vi "SP Retrieve Key Array for Config.vi"(8 "error in (no error)":errorcluster, 9 "Datasheets":T33, 10 "Key Array In":T34, 11 "Connection Refnum":T1) -> (0 "error out":errorcluster, 2 "S Parameter Test Parameters":T2={"Stimulus"={"Use Instrument Settings"=FALSE, "Blank Frequencies"=FALSE, "Sweep Type"=enum."Linear", "Sweep"={"Fstart"=500.0, "Fstop"=1500.0, "Units"=enum."MHz", "Points"=2}, "Power (dBm)"=999.0, "IFBW (Hz)"=-1.0, "Sweep Time (s)"=-1.0, "Calibration"={"State"=FALSE, "String"=""}}, "Measurement"={"Auto Select"=TRUE, "Data Source"=enum."VNA", "Ports"=2, "Parameters"=[]}, "De-Embed"={"De-Embed"=FALSE, "Adapters"=[]}, "Display"={"Lock Control"=FALSE, "Retain Settings"=TRUE, "Formatted Data"=FALSE, "Plot Orientation"=enum."Single", "Plot Controls"=[{"Trace Orientation"=enum."Overlay", "Frequency"={"Change Frequency"=FALSE, "Start"=500.0, "Stop"=1500.0, "Units"=enum."MHz"}, "Markers"=[], "Traces"=[]}, {"Trace Orientation"=enum."Overlay", "Frequency"={"Change Frequency"=FALSE, "Start"=500.0, "Stop"=1500.0, "Units"=enum."MHz"}, "Markers"=[], "Traces"=[]}, {"Trace Orientation"=enum."Overlay", "Frequency"={"Change Frequency"=FALSE, "Start"=500.0, "Stop"=1500.0, "Units"=enum."MHz"}, "Markers"=[], "Traces"=[]}, {"Trace Orientation"=enum."Overlay", "Frequency"={"Change Frequency"=FALSE, "Start"=500.0, "Stop"=1500.0, "Units"=enum."MHz"}, "Markers"=[], "Traces"=[]}]}, "Limits"=[], "Filter Limits"=[]} {"Filter Limits"."Parameter"."Stimulus Port" min=1 step=1; "Filter Limits"."Parameter"."Response Port" min=1 step=1; "Filter Limits"."Passband"."Bandwidth Attn" format="%.3g"; "Filter Limits"."Passband"."Stop/Span" format="%.3g"; "Filter Limits"."Passband"."Start/Center" format="%.3g"; "Measurement"."Parameters"."Channel" min=0 max=32 step=1; "Measurement"."Parameters"."Parameter"."Stimulus Port" min=1 step=1; "Measurement"."Parameters"."Parameter"."Response Port" min=1 step=1; "Limits"."Parameter"."Stimulus Port" min=1 step=1; "Limits"."Parameter"."Response Port" min=1 step=1; "Stimulus"."Sweep Time (s)" format="%.3g"; "Display"."Plot Controls"."Traces"."Reference" format="%#.2g"; "Display"."Plot Controls"."Traces"."Display Data" items=["Data", "Memory", "Data/Memory"]; "Display"."Plot Controls"."Traces"."Format" items=["Log Mag", "Phase", "Expanded Phase", "Delay", "Smith", "Polar", "Lin Mag", "SWR", "Loss", "Real", "Imaginary"]; "Display"."Plot Controls"."Traces"."Scale" min=0.001 step=1.0 format="%#.2g"; "Display"."Plot Controls"."Traces"."Position" min=0.0 max=10.0; "Display"."Plot Controls"."Frequency"."Stop" format="%.3g"; "Display"."Plot Controls"."Frequency"."Start" format="%.3g"}, 3 "Connection Refnum":T1)   [LabVIEW 2011]
uses:
  ITK EXT/utils/keyedarr.llb/Keyed Array.ctl
  Test Datasheets.ctl
  TypeDefs/SP Test Parameters.ctl
  TypeDefs/SP Stimulus Parameters.ctl
  TypeDefs/SP Frequency Units.ctl
  TypeDefs/SP Calibration State.ctl
  TypeDefs/SP Measurement.ctl
  TypeDefs/SP Parameters.ctl
  TypeDefs/SP Parameter.ctl
  TypeDefs/SP De-Embed.ctl
  TypeDefs/SP Adapter.ctl
  TypeDefs/SP Data.ctl
  TypeDefs/SP Display Parameters.ctl
  TypeDefs/SP Display Plot Controls Cluster.ctl
  TypeDefs/SP Marker Cluster.ctl
  TypeDefs/SP Marker Type.ctl
  TypeDefs/SP Display Trace Controls.ctl
  TypeDefs/SP Display Format.ctl
  TypeDefs/SP Display Data.ctl
  TypeDefs/SP Limit.ctl
  TypeDefs/SP Format.ctl
  TypeDefs/SP Limit Type.ctl
  TypeDefs/SP Limit Point.ctl
  Test Referential Limit.ctl
  TypeDefs/SP Filter.ctl
  TypeDefs/SP Filter Type.ctl
  TypeDefs/SP Filter Passband.ctl
  TypeDefs/SP Frequency Format.ctl
  TypeDefs/SP Filter Ripple.ctl
  TypeDefs/SP Attenuation Point.ctl
  TypeDefs/SP Attenuation Type.ctl
  TypeDefs/SP Skirt Rejection Point.ctl
  TypeDefs/SP Relative Loss.ctl
  Summitek EXT/ODBC/SQL Controls/Connection Refnum.ctl
panel:
  # "Div"
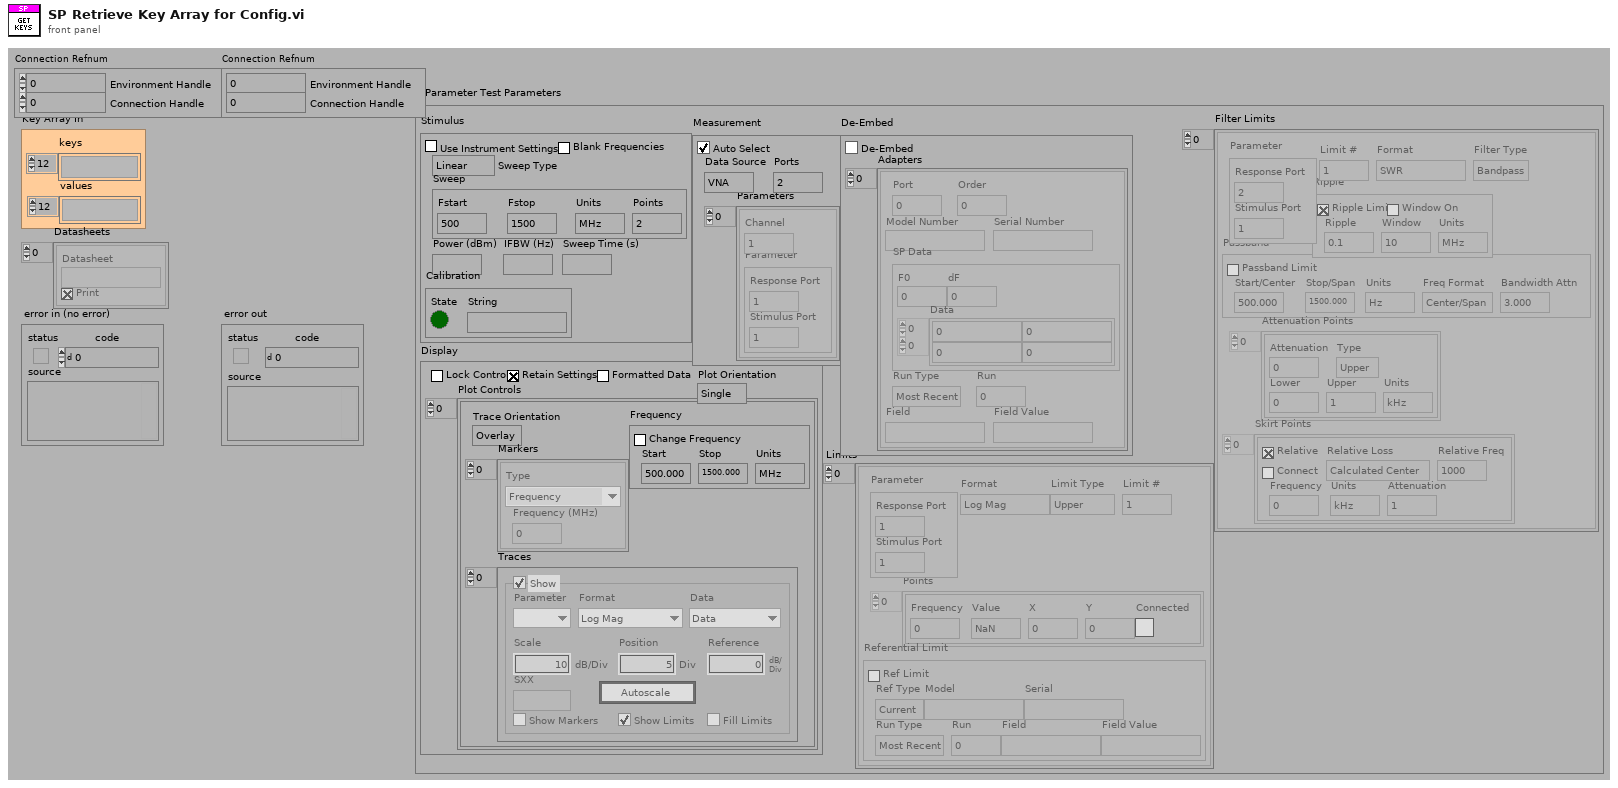
[diagram p1: front panel]
types:
  T1 = typedef "Connection Refnum.ctl" = cluster{"Environment Handle":i32, "Connection Handle":i32}
  T2 = typedef "SP Test Parameters.ctl" = cluster{"Stimulus":T3, "Measurement":T6, "De-Embed":T9, "Display":T12, "Limits":T19[], "Filter Limits":T24[]}
  T3 = typedef "SP Stimulus Parameters.ctl" = cluster{"Use Instrument Settings":bool, "Blank Frequencies":bool, "Sweep Type":enum32{"Linear", "Logarithmic", "List", "Power", "CW"}, "Sweep":cluster{"Fstart":dbl, "Fstop":dbl, "Units":T4, "Points":i32}, "Power (dBm)":dbl, "IFBW (Hz)":dbl, "Sweep Time (s)":dbl, "Calibration":T5}
  T4 = typedef "SP Frequency Units.ctl" = enum16{"Hz", "kHz", "MHz", "GHz", "Points"}
  T5 = typedef "SP Calibration State.ctl" = cluster{"State":bool, "String":string}
  T6 = typedef "SP Measurement.ctl" = cluster{"Auto Select":bool, "Data Source":enum16{"VNA", "Data File"}, "Ports":i8, "Parameters":T7[]}
  T7 = typedef "SP Parameters.ctl" = cluster{"Channel":i8, "Parameter":T8}
  T8 = typedef "SP Parameter.ctl" = cluster{"Stimulus Port":i8, "Response Port":i8}
  T9 = typedef "SP De-Embed.ctl" = cluster{"De-Embed":bool, "Adapters":T10[]}
  T10 = typedef "SP Adapter.ctl" = cluster{"Port":i8, "Order":i8, "Model Number":string, "Serial Number":string, "SP Data":T11, "Run Type":enum16{"Most Recent", "Run #", "Match Field"}, "Run":i32, "Field":string, "Field Value":string}
  T11 = typedef "SP Data.ctl" = cluster{"F0":dbl, "dF":dbl, "Data":cdb[][]}
  T12 = typedef "SP Display Parameters.ctl" = cluster{"Lock Control":bool, "Retain Settings":bool, "Formatted Data":bool, "Plot Orientation":enum32{"Single", "Dual", "Quad"}, "Plot Controls":T13[]}
  T13 = typedef "SP Display Plot Controls Cluster.ctl" = cluster{"Trace Orientation":enum32{"Overlay", "Split"}, "Frequency":cluster{"Change Frequency":bool, "Start":dbl, "Stop":dbl, "Units":T4}, "Markers":T14[], "Traces":T16[]}
  T14 = typedef "SP Marker Cluster.ctl" = cluster{"Type":T15, "Frequency (MHz)":dbl}
  T15 = typedef "SP Marker Type.ctl" = enum16{"Frequency", "Trace Maximum", "Trace Minimum", "Limit Maximum", "Limit Minimum"}
  T16 = typedef "SP Display Trace Controls.ctl" = cluster{"Trace On":bool, "Measure":i32, "Format":T17, "Autoscale":bool, "Reference":dbl, "\nRefUnit":string, "Position":dbl, "Scale":dbl, "ScaleUnit":string, "LimitOn":bool, "LimitFill":bool, "Display Data":T18, "Show Markers":bool, "SXX":string}
  T17 = typedef "SP Display Format.ctl" = i32
  T18 = typedef "SP Display Data.ctl" = u16
  T19 = typedef "SP Limit.ctl" = cluster{"Parameter":T8, "Format":T20, "Limit Type":T21, "Points":T22[], "Referential Limit":T23, "Limit #":i8}
  T20 = typedef "SP Format.ctl" = enum16{"Log Mag", "Lin Mag", "SWR", "Phase", "Expanded Phase", "Delay", "Insertion Loss", "Isolation", "Return Loss"}
  T21 = typedef "SP Limit Type.ctl" = enum16{"Upper", "Lower", "Delta", "Filter", "Referential"}
  T22 = typedef "SP Limit Point.ctl" = cluster{"Frequency":dbl, "Value":dbl, "X":dbl, "Y":dbl, "Connected":bool}
  T23 = typedef "Test Referential Limit.ctl" = cluster{"Ref Limit":bool, "Ref Type":enum16{"Current", "Specify"}, "Model":string, "Serial":string, "Run Type":enum16{"Most Recent", "Run #", "Match Field"}, "Run":i32, "Field":string, "Field Value":string}
  T24 = typedef "SP Filter.ctl" = cluster{"Limit #":i8, "Parameter":T8, "Format":T20, "Filter Type":T25, "Passband":T26, "Ripple":T28, "Attenuation Points":T29[], "Skirt Points":T31[]}
  T25 = typedef "SP Filter Type.ctl" = enum16{"Lowpass", "Highpass", "Bandpass", "Bandstop"}
  T26 = typedef "SP Filter Passband.ctl" = cluster{"Start/Center":dbl, "Stop/Span":dbl, "Units":T4, "Freq Format":T27, "Bandwidth Attn":dbl, "Passband Limit":bool}
  T27 = typedef "SP Frequency Format.ctl" = enum16{"Start/Stop", "Center/Span"}
  T28 = typedef "SP Filter Ripple.ctl" = cluster{"Ripple Limit":bool, "Window On":bool, "Ripple":dbl, "Window":dbl, "Units":T4}
  T29 = typedef "SP Attenuation Point.ctl" = cluster{"Attenuation":dbl, "Type":T30, "Lower":dbl, "Upper":dbl, "Units":T4}
  T30 = typedef "SP Attenuation Type.ctl" = enum16{"Center", "Lower", "Upper"}
  T31 = typedef "SP Skirt Rejection Point.ctl" = cluster{"Relative":bool, "Connect":bool, "Frequency":dbl, "Units":T4, "Attenuation":dbl, "Relative Loss":T32, "Relative Freq":dbl}
  T32 = typedef "SP Relative Loss.ctl" = enum16{"Calculated Center", "Passband Minimum", "Passband Maximum", "Passband Average", "Frequency"}
  T33 = typedef "Test Datasheets.ctl" = cluster{"Datasheet":string, "Print":bool}[]
  T34 = typedef "Keyed Array.ctl" = cluster{"keys":string[], "values":string[]}
  T35 = cluster{"Fstart":dbl, "Fstop":dbl, "Units":T4, "Points":i32}
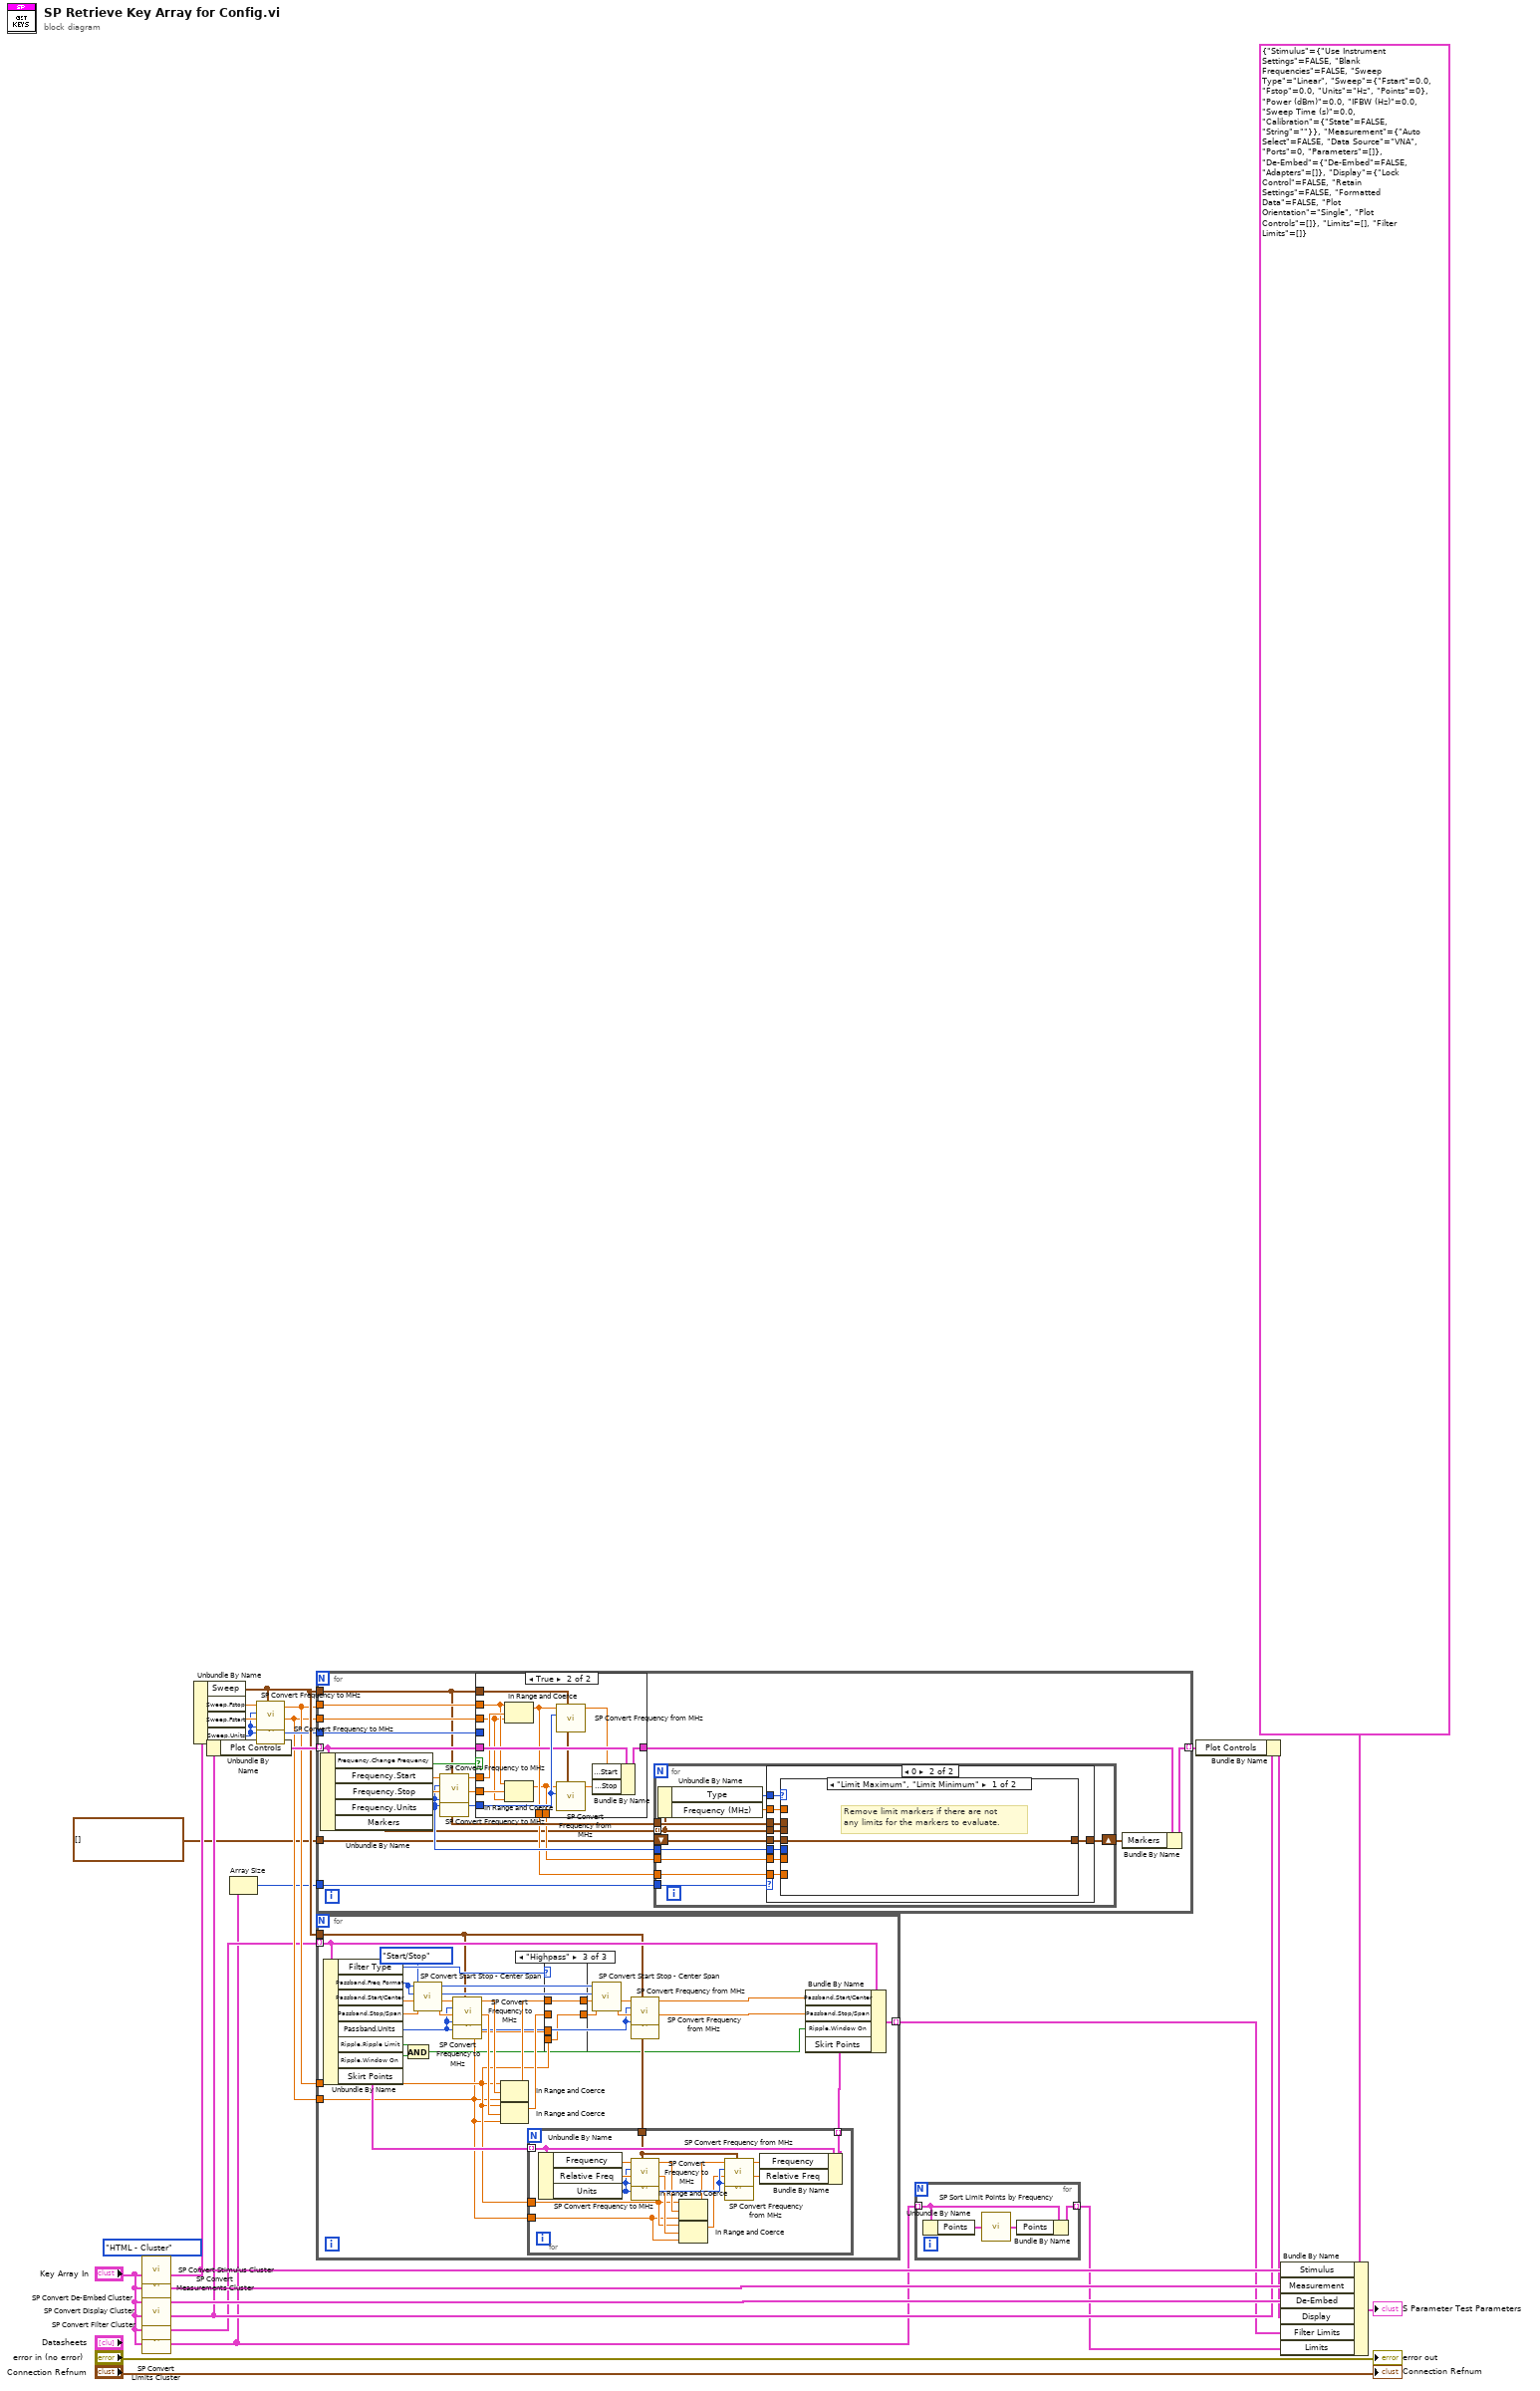
[diagram p0: block diagram]
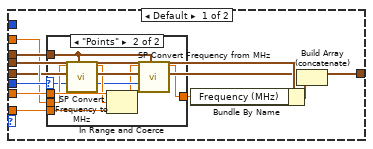
[diagram p4: hidden frame]
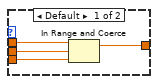
[diagram p5: hidden frame]
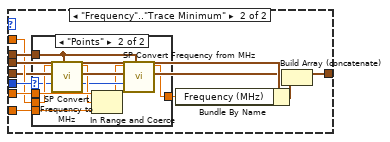
[diagram p6: hidden frame]
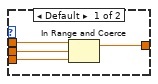
[diagram p7: hidden frame]
diagram:
  w13 = enum16{"Cluster - HTML", "HTML - Cluster"}."HTML - Cluster" ("Conversion")
  n1 = call "SP Convert Stimulus Cluster.vi"("Conversion"=w13, "Stimulus Key Array In"="Key Array In") -> ("Stimulus Cluster Out"=w18:T3)  [unwired: 1 in, 5 out]
  n2 = call "SP Convert Measurements Cluster.vi"("Conversion"=w13, "Measurements Key Array In"="Key Array In") -> ("Measurements Cluster Out"=w22:T6)  [unwired: 1 in, 5 out]
  n3 = call "SP Convert De-Embed Cluster.vi"("Conversion"=w13, "De-Embed Key Array In"="Key Array In") -> ("De-Embed Cluster Out"=w21:T9)  [unwired: 2 in, 5 out]
  n4 = call "SP Convert Display Cluster.vi"("Conversion"=w13, "Display Key Array In"="Key Array In") -> ("Display Cluster Out"=w17:T12)  [unwired: 1 in, 5 out]
  n5 = call "SP Convert Filter Cluster.vi"("Conversion"=w13, "Filter Key Array In"="Key Array In") -> ("Filter Cluster Out"=w6:T24[])  [unwired: 1 in, 6 out]
  n6 = call "SP Convert Limits Cluster.vi"("Conversion"=w13, "Limits Key Array In"="Key Array In") -> ("Limits Cluster Out"=w2:T19[])  [unwired: 2 in, 5 out]
  n7 = Unbundle By Name(w18) -> ("Sweep"=w10:T35, "Sweep.Fstop"=w12:dbl, "Sweep.Fstart"=w11:dbl, "Sweep.Units"=w9:T4)
  n8 = Unbundle By Name(w17) -> ("Plot Controls"=w19:T13[])
  n9 = Array Size(array=w2) -> (size(s)=w4:i32)
  n10 = call "SP Convert Frequency to MHz.vi"("Sweep"=w10, "Units"=w9, "Frequency"=w12) -> ("Converted Frequency"=w8:dbl)  [unwired: 8 out]
  n11 = call "SP Convert Frequency to MHz.vi"("Sweep"=w10, "Units"=w9, "Frequency"=w11) -> ("Converted Frequency"=w7:dbl)  [unwired: 8 out]
  n12 = for {
    tunnel: w19 -> [w43] mode=indexing
    tunnel: [w36] -> w15 mode=indexing
    tunnel: w7 -> [w42]
    tunnel: w8 -> [w41]
    tunnel: w9 -> [w40]
    tunnel: w10 -> [w34]
    tunnel: w4 -> [w29]
    tunnel: T14[] [] ("Markers") -> [w26]
    n13 = Unbundle By Name(w43) -> ("Frequency.Change Frequency"=w44:bool, "Frequency.Start"=w39:dbl, "Frequency.Stop"=w38:dbl, "Frequency.Units"=w35:T4, "Markers"=w28:T14[])
    n14 = call "SP Convert Frequency to MHz.vi"("Sweep"=w34, "Units"=w35, "Frequency"=w39) -> ("Converted Frequency"=w33:dbl)  [unwired: 8 out]
    n15 = call "SP Convert Frequency to MHz.vi"("Sweep"=w34, "Units"=w35, "Frequency"=w38) -> ("Converted Frequency"=w31:dbl)  [unwired: 8 out]
    n16 = case shown="True" w44 {
      tunnel: w43 -> [w111 w122]
      tunnel: [w111 w119] -> w37
      tunnel: w35 -> [_ w123]
      tunnel: w42 -> [_ w112]
      tunnel: w41 -> [_ w113]
      tunnel: w40 -> [_ _]
      tunnel: w34 -> [_ w118]
      tunnel: w31 -> [w109 w117]
      tunnel: w33 -> [w110 w116]
      tunnel: [w110 w115] -> w32
      tunnel: [w109 w114] -> w30
      frame False {
      }
      frame True {
        n17 = In Range and Coerce(upper limit=w113, x=w116, lower limit=w112) -> (coerced(x)=w115:dbl)  [unwired: 1 out]
        n18 = In Range and Coerce(upper limit=w113, x=w117, lower limit=w112) -> (coerced(x)=w114:dbl)  [unwired: 1 out]
        n19 = call "SP Convert Frequency from MHz.vi"("Sweep"=w118, "Units"=w123, "Frequency (MHz)"=w115) -> ("Converted Frequency"=w121:dbl)  [unwired: 8 out]
        n20 = call "SP Convert Frequency from MHz.vi"("Sweep"=w118, "Units"=w123, "Frequency (MHz)"=w114) -> ("Converted Frequency"=w120:dbl)  [unwired: 8 out]
        n21 = Bundle By Name(cluster=w122, "Frequency.Start"=w121, "Frequency.Stop"=w120) -> (w119:T13)
      }
    }
    n22 = for {
      tunnel: w32 -> [w54]
      tunnel: w30 -> [w53]
      tunnel: w35 -> [w52]
      tunnel: w34 -> [w51]
      tunnel: w29 -> [w50]
      shift-right: [w45] -> w27
      shift-left: w26 -> [w46]
      tunnel: w28 -> [w48] mode=indexing
      n23 = Unbundle By Name(w48) -> ("Type"=w49:T15, "Frequency (MHz)"=w47:dbl)
      n24 = case shown="0" w50 {
        tunnel: w54 -> [w64 w85]
        tunnel: w53 -> [w63 w84]
        tunnel: w52 -> [w62 w83]
        tunnel: w51 -> [w61 w82]
        tunnel: w49 -> [_ w81]
        tunnel: w48 -> [w60 w80]
        tunnel: w47 -> [w59 w79]
        tunnel: w46 -> [w56 w78]
        tunnel: [w55 w77] -> w45
        frame Default {
          n25 = case shown="\"Points\"" w62 {
            selector: w62 -> [_ w71]
            tunnel: w64 -> [w68 w76]
            tunnel: w63 -> [w67 w75]
            tunnel: w59 -> [w66 w74]
            tunnel: [w65 w69] -> w58
            tunnel: w61 -> [_ w72]
            frame Default {
              n26 = In Range and Coerce(upper limit=w67, x=w66, lower limit=w68) -> (coerced(x)=w65:dbl)  [unwired: 1 out]
            }
            frame "Points" {
              n27 = call "SP Convert Frequency to MHz.vi"("Sweep"=w72, "Units"=w71, "Frequency"=w74) -> ("Converted Frequency"=w73:dbl)  [unwired: 8 out]
              n28 = In Range and Coerce(upper limit=w75, x=w73, lower limit=w76) -> (coerced(x)=w70:dbl)  [unwired: 1 out]
              n29 = call "SP Convert Frequency from MHz.vi"("Sweep"=w72, "Units"=w71, "Frequency (MHz)"=w70) -> ("Converted Frequency"=w69:dbl)  [unwired: 8 out]
            }
          }
          n30 = Bundle By Name(cluster=w60, "Frequency (MHz)"=w58) -> (w57:T14)
          n31 = Build Array (concatenate)(w56, w57) -> (w55:T14[])
        }
        frame 0 {
          n32 = case shown="\"Limit Maximum\", \"Limit Minimum\"" w81 {
            tunnel: w85 -> [_ w96]
            tunnel: w84 -> [_ w95]
            tunnel: w83 -> [_ w94]
            tunnel: w82 -> [_ w93]
            tunnel: w80 -> [_ w91]
            tunnel: w79 -> [_ w90]
            tunnel: w78 -> [w86 w89]
            tunnel: [w86 w87] -> w77
            frame "Limit Maximum", "Limit Minimum" {
              # "Remove limit markers if there are not\nany limits for the markers to evaluate."
            }
            frame "Frequency".."Trace Minimum" {
              n33 = case shown="\"Points\"" w94 {
                selector: w94 -> [_ w103]
                tunnel: w96 -> [w100 w108]
                tunnel: w95 -> [w99 w107]
                tunnel: w90 -> [w98 w106]
                tunnel: [w97 w101] -> w92
                tunnel: w93 -> [_ w104]
                frame Default {
                  n34 = In Range and Coerce(upper limit=w99, x=w98, lower limit=w100) -> (coerced(x)=w97:dbl)  [unwired: 1 out]
                }
                frame "Points" {
                  n35 = call "SP Convert Frequency to MHz.vi"("Sweep"=w104, "Units"=w103, "Frequency"=w106) -> ("Converted Frequency"=w105:dbl)  [unwired: 8 out]
                  n36 = In Range and Coerce(upper limit=w107, x=w105, lower limit=w108) -> (coerced(x)=w102:dbl)  [unwired: 1 out]
                  n37 = call "SP Convert Frequency from MHz.vi"("Sweep"=w104, "Units"=w103, "Frequency (MHz)"=w102) -> ("Converted Frequency"=w101:dbl)  [unwired: 8 out]
                }
              }
              n38 = Bundle By Name(cluster=w91, "Frequency (MHz)"=w92) -> (w88:T14)
              n39 = Build Array (concatenate)(w89, w88) -> (w87:T14[])
            }
          }
        }
      }
    }
    n40 = Bundle By Name(cluster=w37, "Markers"=w27) -> (w36:T13)
  }
  n41 = for {
    tunnel: w6 -> [w151] mode=indexing
    tunnel: w10 -> [w130]
    tunnel: w8 -> [w129]
    tunnel: w7 -> [w128]
    tunnel: [w132] -> w5 mode=indexing
    n42 = Unbundle By Name(w151) -> ("Filter Type"=w152:T25, "Passband.Freq Format"=w134:T27, "Passband.Start/Center"=w145:dbl, "Passband.Stop/Span"=w143:dbl, "Passband.Units"=w135:T4, "Ripple.Ripple Limit"=w125:bool, "Ripple.Window On"=w126:bool, "Skirt Points"=w131:T31[])
    n43 = And(x=w125, y=w126) -> (x .and. y?=w124:bool)
    n44 = call "SP Convert Start Stop - Center Span.vi"("Stop/Span In"=w143, "Start/Center In"=w145, "Freq Format From"=w134, "Freq Format To"=SP_Frequency_Format."Start/Stop") -> ("Stop/Span Out"=w142:dbl, "Start/Center Out"=w144:dbl, "Freq Format"=w133:T27)  [unwired: 5 out]
    n45 = call "SP Convert Frequency to MHz.vi"("Sweep"=w130, "Units"=w135, "Frequency"=w144) -> ("Converted Frequency"=w150:dbl)  [unwired: 8 out]
    n46 = call "SP Convert Frequency to MHz.vi"("Sweep"=w130, "Units"=w135, "Frequency"=w142) -> ("Converted Frequency"=w148:dbl)  [unwired: 8 out]
    n47 = In Range and Coerce(upper limit=w129, x=w150, lower limit=w128) -> (coerced(x)=w149:dbl)  [unwired: 1 out]
    n48 = In Range and Coerce(upper limit=w129, x=w148, lower limit=w128) -> (coerced(x)=w147:dbl)  [unwired: 1 out]
    n49 = for {
      tunnel: w131 -> [w165] mode=indexing
      tunnel: w130 -> [w160]
      tunnel: w129 -> [w155]
      tunnel: w128 -> [w154]
      tunnel: [w153] -> w127 mode=indexing
      n50 = Unbundle By Name(w165) -> ("Frequency"=w166:dbl, "Relative Freq"=w163:dbl, "Units"=w161:T4)
      n51 = call "SP Convert Frequency to MHz.vi"("Sweep"=w160, "Units"=w161, "Frequency"=w166) -> ("Converted Frequency"=w158:dbl)  [unwired: 8 out]
      n52 = call "SP Convert Frequency to MHz.vi"("Sweep"=w160, "Units"=w161, "Frequency"=w163) -> ("Converted Frequency"=w159:dbl)  [unwired: 8 out]
      n53 = In Range and Coerce(upper limit=w155, x=w158, lower limit=w154) -> (coerced(x)=w157:dbl)  [unwired: 1 out]
      n54 = In Range and Coerce(upper limit=w155, x=w159, lower limit=w154) -> (coerced(x)=w156:dbl)  [unwired: 1 out]
      n55 = call "SP Convert Frequency from MHz.vi"("Sweep"=w160, "Units"=w161, "Frequency (MHz)"=w157) -> ("Converted Frequency"=w164:dbl)  [unwired: 8 out]
      n56 = call "SP Convert Frequency from MHz.vi"("Sweep"=w160, "Units"=w161, "Frequency (MHz)"=w156) -> ("Converted Frequency"=w162:dbl)  [unwired: 8 out]
      n57 = Bundle By Name(cluster=w165, "Frequency"=w164, "Relative Freq"=w162) -> (w153:T31)
    }
    n58 = case shown="\"Highpass\"" w152 {
      tunnel: w149 -> [w168 _ w172]
      tunnel: w147 -> [w167 w170 _]
      tunnel: w129 -> [_ _ w171]
      tunnel: w128 -> [_ w169 _]
      tunnel: [w168 w169 w172] -> w141
      tunnel: [w167 w170 w171] -> w140
      frame "Bandpass", "Bandstop" {
      }
      frame "Lowpass" {
      }
      frame "Highpass" {
      }
    }
    n59 = call "SP Convert Start Stop - Center Span.vi"("Stop/Span In"=w140, "Start/Center In"=w141, "Freq Format From"=w133, "Freq Format To"=w134) -> ("Stop/Span Out"=w136:dbl, "Start/Center Out"=w138:dbl)  [unwired: 6 out]
    n60 = call "SP Convert Frequency from MHz.vi"("Sweep"=w130, "Units"=w135, "Frequency (MHz)"=w138) -> ("Converted Frequency"=w139:dbl)  [unwired: 8 out]
    n61 = call "SP Convert Frequency from MHz.vi"("Sweep"=w130, "Units"=w135, "Frequency (MHz)"=w136) -> ("Converted Frequency"=w137:dbl)  [unwired: 8 out]
    n62 = Bundle By Name(cluster=w151, "Passband.Start/Center"=w139, "Passband.Stop/Span"=w137, "Ripple.Window On"=w124, "Skirt Points"=w127) -> (w132:T24)
  }
  n63 = for {
    tunnel: w2 -> [w175] mode=indexing
    tunnel: [w173] -> w1 mode=indexing
    n64 = Unbundle By Name(w175) -> ("Points"=w176:T22[])
    n65 = call "SP Sort Limit Points by Frequency.vi"("Points"=w176) -> ("Sorted Points"=w174:T22[])  [unwired: 4 out]
    n66 = Bundle By Name(cluster=w175, "Points"=w174) -> (w173:T19)
  }
  n67 = Bundle By Name(cluster=w17, "Plot Controls"=w15) -> (w16:T12)
  n68 = Bundle By Name(cluster=T2 {"Stimulus"={"Use Instrument Settings"=FALSE, "Blank Frequencies"=FALSE, "Sweep Type"=enum."Linear", "Sweep"={"Fstart"=0.0, "Fstop"=0.0, "Units"=enum."Hz", "Points"=0}, "Power (dBm)"=0.0, "IFBW (Hz)"=0.0, "Sweep Time (s)"=0.0, "Calibration"={"State"=FALSE, "String"=""}}, "Measurement"={"Auto Select"=FALSE, "Data Source"=enum."VNA", "Ports"=0, "Parameters"=[]}, "De-Embed"={"De-Embed"=FALSE, "Adapters"=[]}, "Display"={"Lock Control"=FALSE, "Retain Settings"=FALSE, "Formatted Data"=FALSE, "Plot Orientation"=enum."Single", "Plot Controls"=[]}, "Limits"=[], "Filter Limits"=[]} ("S Parameter Test Parameters"), "Stimulus"=w18, "Measurement"=w22, "De-Embed"=w21, "Display"=w16, "Filter Limits"=w5, "Limits"=w1) -> (→"S Parameter Test Parameters":T2)
  "error out" <- "error in (no error)"
  "Connection Refnum" <- "Connection Refnum"
